vi "niHWS Write Digital 2D U8.vi"(8 "error in (no error)":errorcluster, 10 "data":u8[][](array[numeric]), 11 "waveform reference in":u32) -> (0 "error out":errorcluster, 3 "waveform reference out":u32)   [LabVIEW 2013]
doc: "Writes a two-dimensional array of 8-bit unsigned integer (U8) digital waveform data into the file beginning at the current read/write position."
uses:
  nihwsu.dll
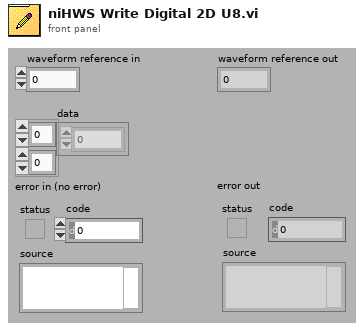
[diagram p1: front panel]
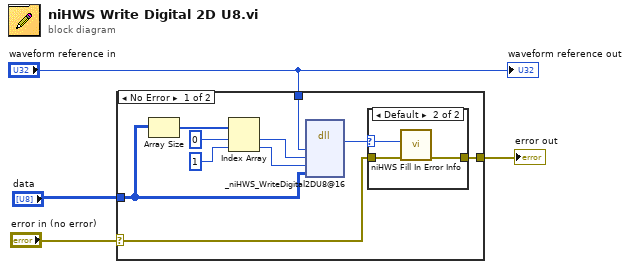
[diagram p0: block diagram]
diagram:
  n1 = case shown="No Error" "error in (no error)" {
    selector: "error in (no error)" -> [w12 w19]
    tunnel: [w13 w19] -> w3
    tunnel: "waveform reference in" -> [w14 _]
    tunnel: "data" -> [w5 _]
    frame No Error {
      n2 = Array Size(array=w5) -> (size(s)=w10:i32[])
      n3 = Index Array(array=w10, index #1=0 ("index"), index #2=1 ("index")) -> (element #1=w7:i32, element #2=w6:i32)
      n4 = dll-call lib="nihwsu.dll" fn="_niHWS_WriteDigital2DU8@16"("wfmReference"=w14, "numRows"=w7, "numSamples"=w6, "wfmData"=w5) -> (w11:i32)  [unwired: 7 in, 2 out]
      n5 = case shown="Default" w11 {
        selector: w11 -> [_ w16]
        tunnel: [w15 w17] -> w13
        tunnel: w12 -> [w15 w18]
        frame 0 {
        }
        frame Default {
          n6 = call "niHWS Fill In Error Info.vi"("error in (no error)"=w18, "status code"=w16) -> ("error out"=w17:errorcluster)  [unwired: 9 in]
        }
      }
    }
    frame Error {
    }
  }
  "error out" <- w3
  "waveform reference out" <- "waveform reference in"
